vi "Renishaw-XL80_GetMl10Status.vi"(8 "error in (no error)":errorcluster, 11 "Renishaw-XL80_EMU in":refnum<class "Renishaw-XL80_EMU.lvclass">) -> (0 "error out":errorcluster, 2 "ML10Status":i32(ring)=1 items=["ML10_AVERAGING_ON"=1, "ML10_TPIN_SELECTED"=4, "ML10_BEAM_LOW"=64, "ML10_BEAM_LOSS"=128, "ML10_STABILITY_LOSS"=256, "ML10_PREHEAT"=2048, "ML10_LASER_TOO_COLD"=4096, "ML10_LASER_TOO_HOT"=8192, "ML10_LASER_UNSTABLE"=16384, "ML10_LASER_FAIL"=32768, "ML10_NOT_RESPONDING"=65536, "ML10_LONG_TERM_AVERAGING_ON"=524288, "ML10_MEASUREMENT_MODE"=7340032, "ML10_HIGH_SPEED_ERROR"=8388608, "ML10_DYNAMIC_SELECTED"=16777216], 3 "Renishaw-XL80_EMU out":refnum<class "Renishaw-XL80_EMU.lvclass">)   [LabVIEW 2024, in "Renishaw-XL80_EMU.lvclass"]
doc: "This read only property returns the current status of the ML10.\n\nDefinition\nHRESULTget_ML10Status( [out, retval] ML10_STATUS_CODES* pVal);\nParameters\npVal\nA variable that will be set to ML10_STATUS_CODES.\n\nComments\nThis property will return with an HRESULT of E_FAIL if the client has not previously connected to a DX10 by calling Connect.\n\nIf the client has connected then this property will normally return an HRESULT of S_OK. However, it will return E_POINTER if the client supplies a null pointer for pVal.\n\nNote: if there is a XL laser connected to the DX10Adaptor COM interface then this property returns the XL laser's status"
uses:
  Renishaw-XL80_EMU.lvclass
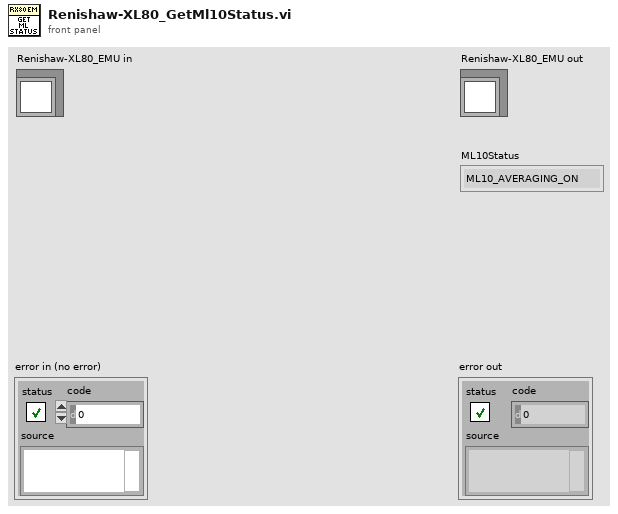
[diagram p1: front panel]
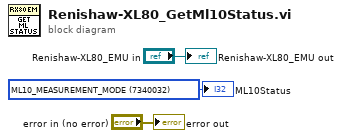
[diagram p0: block diagram]
diagram:
  w1 = 7340032 items=["ML10_AVERAGING_ON"=1, "ML10_TPIN_SELECTED"=4, "ML10_BEAM_LOW"=64, "ML10_BEAM_LOSS"=128, "ML10_STABILITY_LOSS"=256, "ML10_PREHEAT"=2048, "ML10_LASER_TOO_COLD"=4096, "ML10_LASER_TOO_HOT"=8192, "ML10_LASER_UNSTABLE"=16384, "ML10_LASER_FAIL"=32768, "ML10_NOT_RESPONDING"=65536, "ML10_LONG_TERM_AVERAGING_ON"=524288, "ML10_MEASUREMENT_MODE"=7340032, "ML10_HIGH_SPEED_ERROR"=8388608, "ML10_DYNAMIC_SELECTED"=16777216] ("ML10Status")
  "error out" <- "error in (no error)"
  "Renishaw-XL80_EMU out" <- "Renishaw-XL80_EMU in"
  "ML10Status" <- w1
